vi "4155C QSCV Config SMUs.vi"(0 "VISA resource name in":refnum<visa-resource-name>, 2 "Gate mode":u16(ring) items=["Auto", "Limited", "Fixed"], 3 "Gate Range":u8(slide)=6 max=11 scale=0.0..11.0, 11 "error in (no error)":errorcluster, 13 "Source/drain mode":u16(ring) items=["Auto", "Limited", "Fixed"], 14 "Source/drain Range":u8(slide)=6 max=11 scale=0.0..11.0) -> (4 "VISA Resource Name out":refnum<visa-resource-name>, 15 "error out":errorcluster)   [LabVIEW 2016]
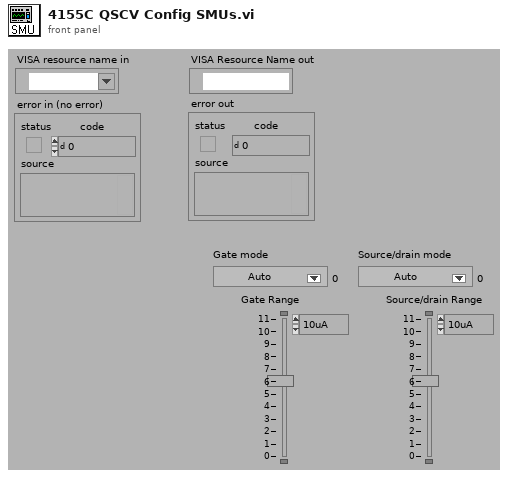
[diagram p1: front panel]
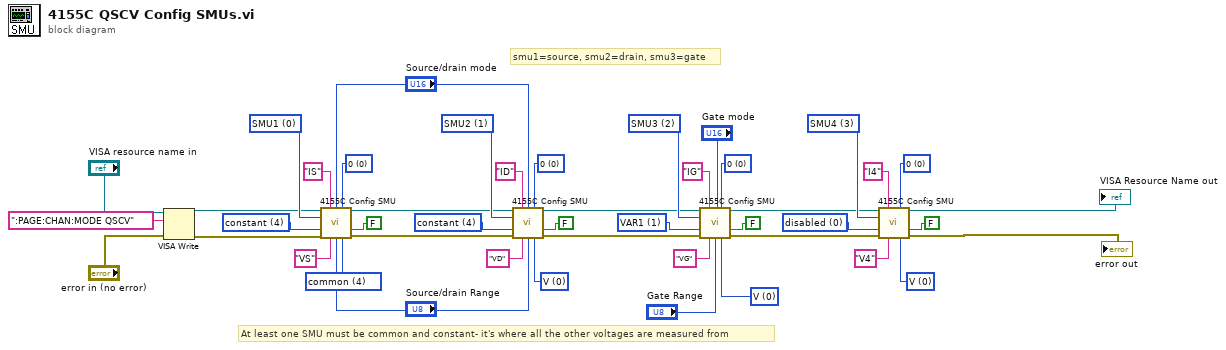
[diagram p0: block diagram]
diagram:
  w8 = u32 0 items=["V  ", "I  ", "V pulse  ", "I pulse  ", "  common  "] ("mode")
  w21 = u32 0 items=["V  ", "I  ", "V pulse  ", "I pulse  ", "  common  "] ("mode")
  w22 = u32 0 items=["0  ", "10K Ohms  ", "100K Ohms  ", "1M Ohms  "] ("series resistance *")
  w24 = u32 0 items=["disabled  ", "VAR1  ", "VAR2  ", "VAR1'  ", "constant  "] ("function")
  w25 = u32 3 items=["SMU1  ", "SMU2  ", "SMU3  ", "SMU4  ", "SMU5  ", "SMU6  "] ("unit to configure")
  w28 = u32 0 items=["0  ", "10K Ohms  ", "100K Ohms  ", "1M Ohms  "] ("series resistance *")
  w30 = u32 1 items=["disabled  ", "VAR1  ", "VAR2  ", "VAR1'  ", "constant  "] ("function")
  w31 = u32 2 items=["SMU1  ", "SMU2  ", "SMU3  ", "SMU4  ", "SMU5  ", "SMU6  "] ("unit to configure")
  w34 = u32 0 items=["V  ", "I  ", "V pulse  ", "I pulse  ", "  common  "] ("mode")
  w35 = u32 0 items=["0  ", "10K Ohms  ", "100K Ohms  ", "1M Ohms  "] ("series resistance *")
  w37 = u32 4 items=["disabled  ", "VAR1  ", "VAR2  ", "VAR1'  ", "constant  "] ("function")
  w38 = u32 1 items=["SMU1  ", "SMU2  ", "SMU3  ", "SMU4  ", "SMU5  ", "SMU6  "] ("unit to configure")
  w41 = u32 4 items=["V  ", "I  ", "V pulse  ", "I pulse  ", "  common  "] ("mode")
  w42 = u32 0 items=["0  ", "10K Ohms  ", "100K Ohms  ", "1M Ohms  "] ("series resistance *")
  w44 = u32 4 items=["disabled  ", "VAR1  ", "VAR2  ", "VAR1'  ", "constant  "] ("function")
  w45 = u32 0 items=["SMU1  ", "SMU2  ", "SMU3  ", "SMU4  ", "SMU5  ", "SMU6  "] ("unit to configure")
  # "smu1=source, smu2=drain, smu3=gate"
  # "At least one SMU must be common and constant- it's where all the other voltages are measured from"
  n1 = VISA Write(VISA resource name="VISA resource name in", write buffer=":PAGE:CHAN:MODE QSCV" ("write buffer (\"\")"), error in (no error)="error in (no error)") -> (VISA resource name out=w6:refnum<visa-resource-name>, error out=w7:errorcluster)  [unwired: 1 out]
  n2 = call "4155C Config SMU.vi"("VISA session"=w6, "I name (max 6 chars)"="IS", "Range mode"="Source/drain mode", "series resistance *"=w42, "unit to configure"=w45, "function"=w44, "standby"=FALSE, "error in (no error)"=w7, "V name (max 6 chars)"="VS", "Range"="Source/drain Range", "mode"=w41) -> ("dup VISA resource name"=w18:refnum<visa-resource-name>, "error out"=w17:errorcluster)  [unwired: 3 in]
  n3 = call "4155C Config SMU.vi"("VISA session"=w18, "I name (max 6 chars)"="ID", "Range mode"="Source/drain mode", "series resistance *"=w35, "unit to configure"=w38, "function"=w37, "standby"=FALSE, "error in (no error)"=w17, "V name (max 6 chars)"="VD", "Range"="Source/drain Range", "mode"=w34) -> ("dup VISA resource name"=w15:refnum<visa-resource-name>, "error out"=w16:errorcluster)  [unwired: 3 in]
  n4 = call "4155C Config SMU.vi"("VISA session"=w15, "I name (max 6 chars)"="IG", "Range mode"="Gate mode", "series resistance *"=w28, "unit to configure"=w31, "function"=w30, "standby"=FALSE, "error in (no error)"=w16, "V name (max 6 chars)"="VG", "Range"="Gate Range", "mode"=w8) -> ("dup VISA resource name"=w14:refnum<visa-resource-name>, "error out"=w13:errorcluster)  [unwired: 3 in]
  n5 = call "4155C Config SMU.vi"("VISA session"=w14, "I name (max 6 chars)"="I4", "series resistance *"=w22, "unit to configure"=w25, "function"=w24, "standby"=FALSE, "error in (no error)"=w13, "V name (max 6 chars)"="V4", "mode"=w21) -> ("dup VISA resource name"=→"VISA Resource Name out":refnum<visa-resource-name>, "error out"=→"error out":errorcluster)  [unwired: 5 in]
